vi "Write BoolText.vi"(5 "BoolText":refnum<class "Text.lvclass">, 9 "Boolean in":refnum<class "Boolean.lvclass">) -> (3 "Boolean out":refnum<class "Boolean.lvclass">)   [LabVIEW 2014, in "Boolean.lvclass"]
uses:
  Boolean.lvclass
  Text/Text.lvclass
  Boolean.lvclass/Boolean.ctl
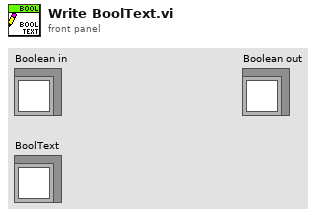
[diagram p1: front panel]
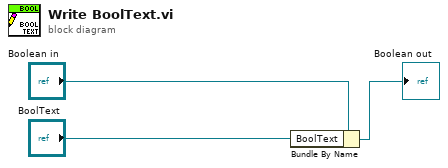
[diagram p0: block diagram]
diagram:
  n1 = Bundle By Name(cluster="Boolean in", "BoolText"="BoolText") -> (→"Boolean out":refnum<class "Boolean.lvclass">)
